vi "Configure Offset and Limits (Adjacent Channel Power - Offset Frequency and Integration Bandwidth).vi"(0 "VISA resource name":refnum<visa-resource-name>, 1 "Offset Integration Bandwidth List":dbl[](array[numeric])=[2000000.0, 2000000.0, 2000000.0, 2000000.0, 2000000.0, 2000000.0], 5 "Device Mode (1: BTS)":i32(ring)=1 items=["BTS"=1, "MS"=2], 7 "Offset Frequency List":dbl[](array[numeric])=[3000000.0, 3000000.0, 3000000.0, 3000000.0, 3000000.0, 3000000.0], 9 "Enable Offset Frequency List":bool[](array[boolean])=[FALSE, FALSE, FALSE, FALSE, FALSE, FALSE], 11 "error in (no error)":errorcluster) -> (4 "VISA resource name out":refnum<visa-resource-name>, 15 "error out":errorcluster)   [LabVIEW 2014, in "Agilent MXA Series.lvlib"]
doc: "Configures the offset frequency under the offsets and limits for ACP measurement type."
uses:
  Agilent MXA Series.lvlib
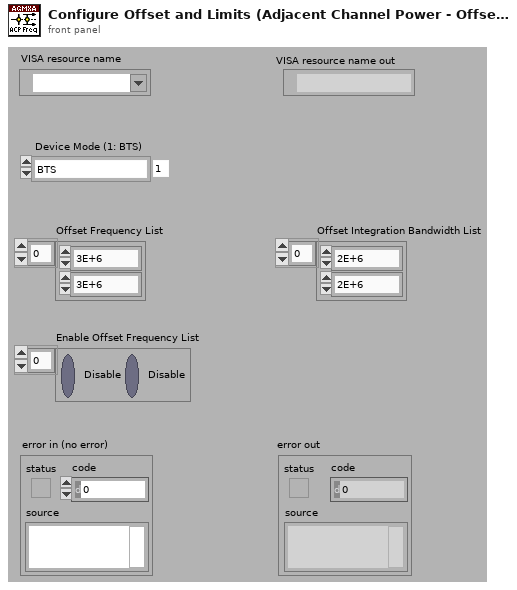
[diagram p1: front panel]
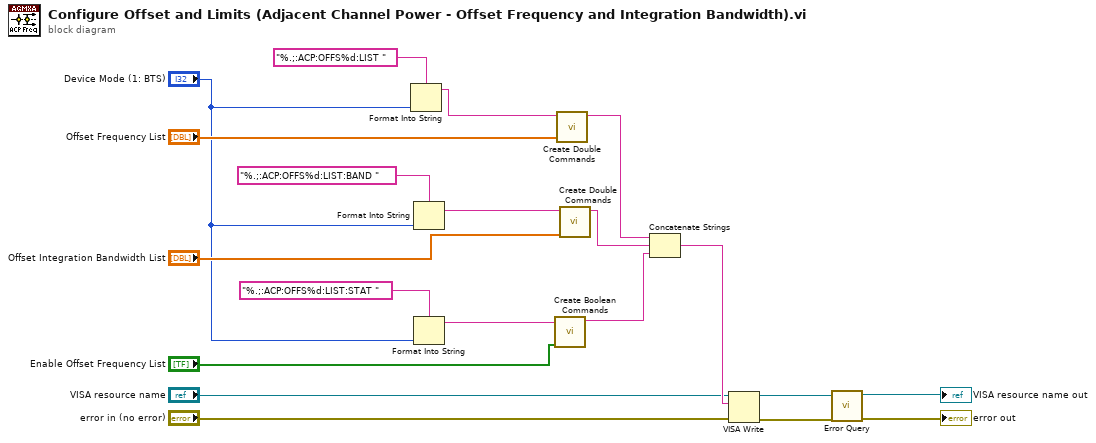
[diagram p0: block diagram]
diagram:
  n1 = Format Into String(format string="%.;:ACP:OFFS%d:LIST ", "Device Mode (1: BTS)") -> (resulting string=w19:string)  [unwired: 2 in, 1 out]
  n2 = Format Into String(format string="%.;:ACP:OFFS%d:LIST:BAND ", "Device Mode (1: BTS)") -> (resulting string=w16:string)  [unwired: 2 in, 1 out]
  n3 = Format Into String(format string="%.;:ACP:OFFS%d:LIST:STAT ", "Device Mode (1: BTS)") -> (resulting string=w13:string)  [unwired: 2 in, 1 out]
  n4 = call "Create Boolean Commands.vi"("Boolean States"="Enable Offset Frequency List", "Command"=w13) -> ("Result String"=w7:string)  [unwired: 9 in]
  n5 = call "Create Double Commands.vi"("Double Values"="Offset Frequency List", "Commands"=w19) -> ("Result"=w9:string)  [unwired: 9 in]
  n6 = call "Create Double Commands.vi"("Double Values"="Offset Integration Bandwidth List", "Commands"=w16) -> ("Result"=w8:string)  [unwired: 9 in]
  n7 = Concatenate Strings(w9, w8, w7) -> (w6:string)
  n8 = VISA Write(VISA resource name="VISA resource name", write buffer=w6, error in (no error)="error in (no error)") -> (VISA resource name out=w10:refnum<visa-resource-name>, error out=w11:errorcluster)  [unwired: 1 out]
  n9 = call "Error Query.vi"("error in (no error)"=w11, "VISA resource name"=w10) -> ("error out"=→"error out":errorcluster, "VISA resource name out"=→"VISA resource name out":refnum<visa-resource-name>)  [unwired: 6 in, 2 out]
